vi "Main.vi"() -> ()   [LabVIEW 2015, in "Stock.lvlib"]
doc: "This template is based off of the Queued Message Handler design pattern and the Queued Message Handler project template that ships with LabVIEW.\n\nThe main difference is that the queue is private to this module and communication between modules is performed via Broadcast and Request events.\n\nRequest events are wrapped in public API methods and are handled in the Event Handling Loop (EHL) of this VI. Any module can register for Broadcast events sent by this module. The EHL generates messages based on user interface actions.\n\nThe Message Handling Loop (MHL) processes messages generated by the EHL, or by other messages. The messages are string values, so new messages can be added easily to the Message Cases case structure in the MHL. Each message cluster can also provide an optional value for Message Data, which is a variant that can be converted to whatever message-specific data is required.\n_____\nBased on Delacor QMH Project Template 4.2.1.64."
uses:
  Stock.lvlib
  <vilib>/Delacor/Delacor QMH/Libraries/Module Admin_class/Delacor_lib_QMH_Module Admin.lvclass
  Module Data--cluster.ctl
  Products.ctl
  <vilib>/Delacor/Delacor QMH/Libraries/Message Queue_class/Delacor_lib_QMH_Message Queue.lvclass/Delacor_lib_QMH_Message Queue.ctl
  Stop Argument--cluster.ctl
  <vilib>/Delacor/Delacor QMH/Libraries/Module Admin_class/Delacor_lib_QMH_Module Admin.lvclass/Delacor_lib_QMH_Module Admin.ctl
  In Stock and Price Argument--cluster.ctl
  In Stock and Price (Reply Payload)--cluster.ctl
  Reduce Stock Level Argument--cluster.ctl
  Reduce Stock Level (Reply Payload)--cluster.ctl
  <vilib>/Utility/miscctls.llb/LVPointTypeDef.ctl
  <vilib>/Delacor/Delacor QMH/Libraries/Message Queue_class/Delacor_lib_QMH_Enqueue Message (Single).vi
  <vilib>/Delacor/Delacor QMH/Libraries/Module Admin_class/Delacor_lib_QMH_Get External Launch.vi
  <vilib>/Utility/error.llb/Error Cluster From Error Code.vi
  <vilib>/ErrorRing/Error Ring.xnode
  <vilib>/Delacor/Delacor QMH/Libraries/Message Queue_class/Delacor_lib_QMH_Message Queue.lvclass
panel:
  in  "Subpanel Ref":refnum<vi>
  out "Stock Levels":T1(array[cluster]) {"Price" format="£%.2f"; "Stock Level" scale=0.0..58.0}
  in  "Simulate MHL Error":bool
  in  "Simulate EHL Error":bool
  out "error out":errorcluster
  in  "Module Admin":refnum<class "Delacor_lib_QMH_Module Admin.lvclass">
  out "Status":string
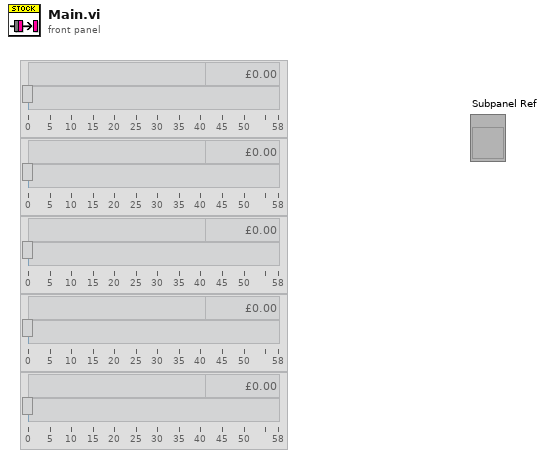
[diagram p1: front panel]
types:
  T1 = cluster{"Name":string, "Price":dbl, "Stock Level":dbl}[]
  T2 = typedef "Stock.lvlib/Request Events--cluster.ctl" = cluster{"Stop Module":refnum<user-event>, "Show Panel":refnum<user-event>, "Hide Panel":refnum<user-event>, "Get Module Execution Status":refnum<user-event>, "Show Diagram":refnum<user-event>, "In Stock and Price":refnum<user-event>, "Reduce Stock Level":refnum<user-event>}
  T3 = typedef "Stock.lvlib/Module Data--cluster.ctl" = cluster{"Status":string, "Stock":T4[], "Stock File Path":path}
  T4 = typedef "Stock.lvlib/Products.ctl" = cluster{"Name":string, "Price (pence/cents)":u32, "Stock Level":u32}
  T5 = enum32{"invalid lock state", "Not Locked", "Locked (No Password)", "Password-protected"}
  T6 = typedef "Stock.lvlib/Stop Argument--cluster.ctl" = cluster{"Origin":string, "Exit via Stop Module Req?":bool, "Wait for Module to stop?":bool}
  T7 = typedef "Stock.lvlib/In Stock and Price Argument--cluster.ctl" = cluster{"Stock Item":u32, "Wait Notifier":refnum<notifier>, "wait for reply":bool}
  T8 = typedef "Stock.lvlib/Reduce Stock Level Argument--cluster.ctl" = cluster{"Product":i32, "Wait Notifier":refnum<notifier>, "wait for reply":bool}
  T9 = typedef "LVPointTypeDef.ctl" = cluster{"Horizontal":i16, "Vertical":i16}
  T10 = typedef "Stock.lvlib/In Stock and Price (Reply Payload)--cluster.ctl" = cluster{"In Stock?":bool, "Price (Pence)":u32, "In Stock and Price_error":errorcluster}
  T11 = typedef "Stock.lvlib/Reduce Stock Level (Reply Payload)--cluster.ctl" = cluster{"Sucessful?":bool, "Reduce Stock Level_error":errorcluster}
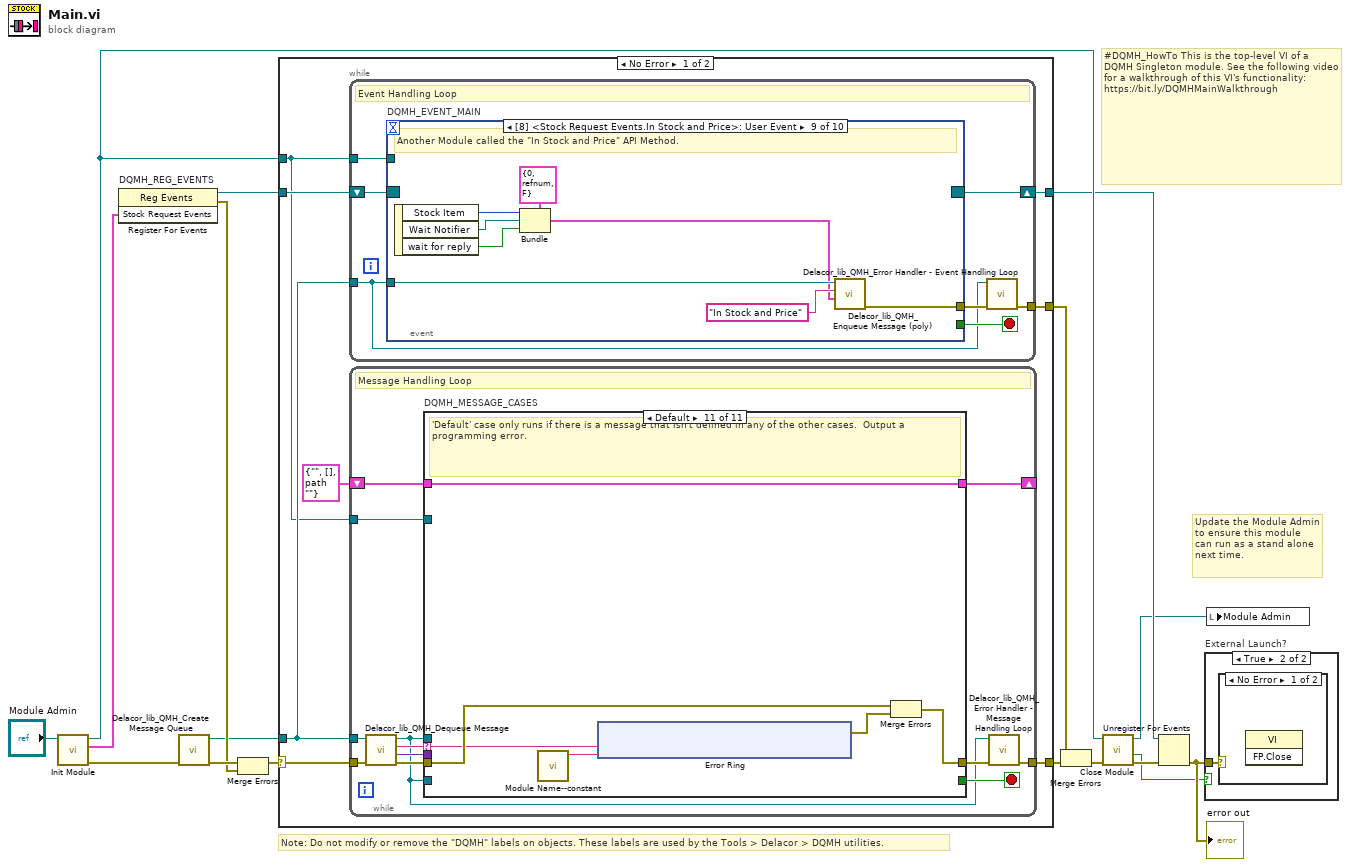
[diagram p0: block diagram]
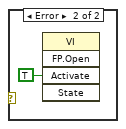
[diagram p3: hidden frame]
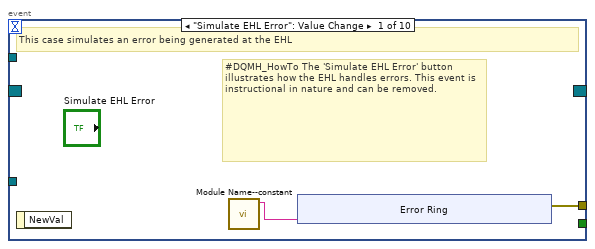
[diagram p4: hidden frame]
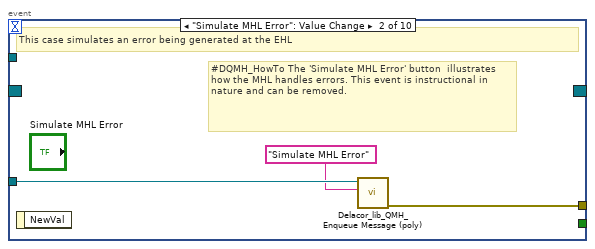
[diagram p5: hidden frame]
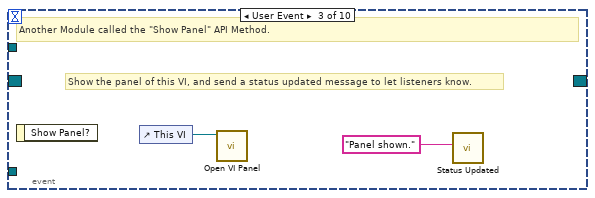
[diagram p6: hidden frame]
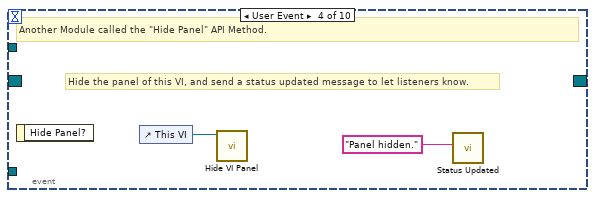
[diagram p7: hidden frame]
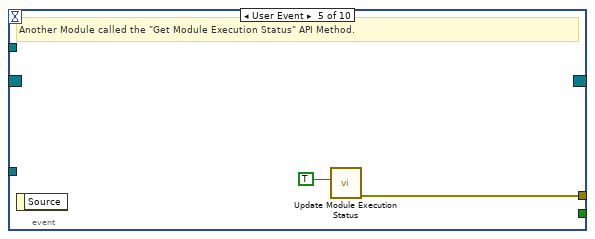
[diagram p8: hidden frame]
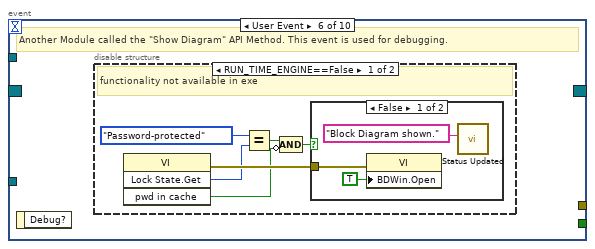
[diagram p9: hidden frame]
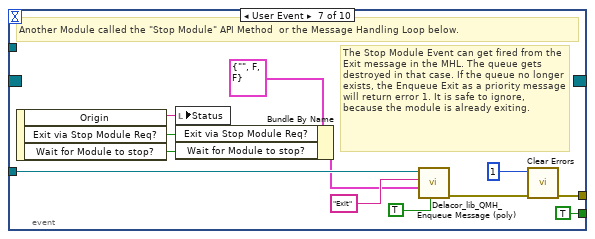
[diagram p12: hidden frame]
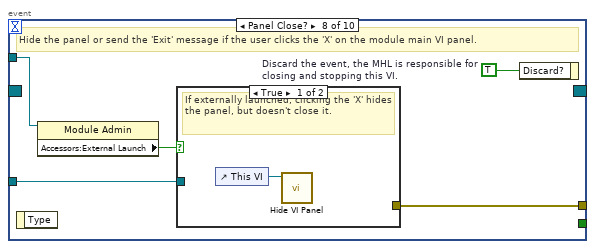
[diagram p13: hidden frame]
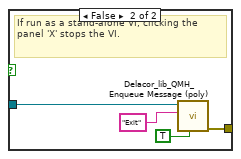
[diagram p14: hidden frame]
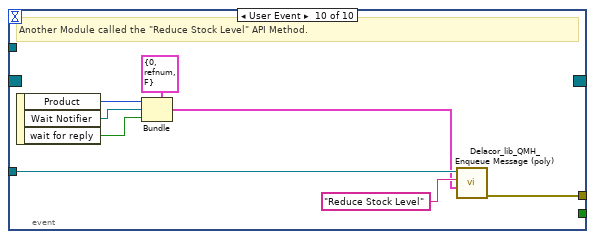
[diagram p15: hidden frame]
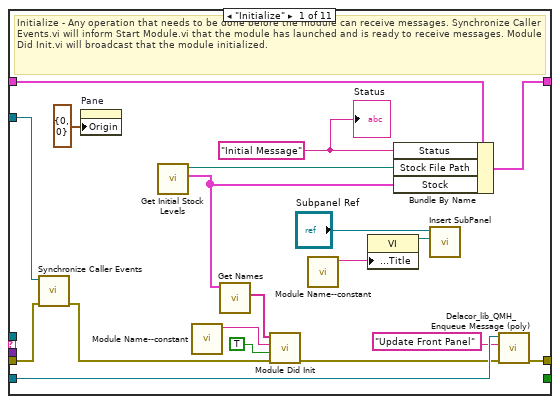
[diagram p16: hidden frame]
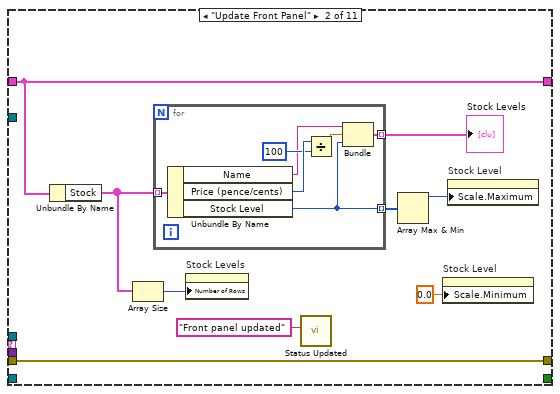
[diagram p17: hidden frame]
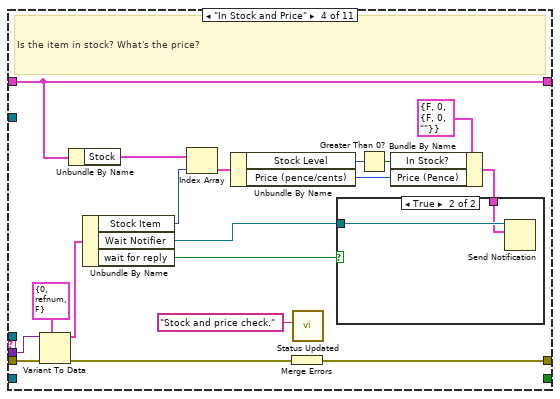
[diagram p19: hidden frame]
diagram:
  # "#DQMH_HowTo This is the top-level VI of a DQMH Singleton module. See the following video for a walkthrough of this VI's functionality: https://bit.ly/DQMHMainWalkthrough"
  # "Note: Do not modify or remove the \"DQMH\" labels on objects. These labels are used by the Tools > Delacor > DQMH utilities."
  # "Update the Module Admin to ensure this module can run as a stand alone next time."
  n1 = call "Init Module.vi"("Singleton Module Admin in"="Module Admin") -> ("error out"=w16:errorcluster, "Stock Request Events"=w5:T2, "Singleton Module Admin out"=w8:refnum<class "Delacor_lib_QMH_Module Admin.lvclass">)  [unwired: 8 in]
  n2 = register-events "DQMH_REG_EVENTS"(w5) -> (reference out=w6:refnum<event-registration>, error out=w9:errorcluster)  [unwired: 2 in]
  n3 = call <vilib>:"Delacor_lib_QMH_Create Message Queue.vi"("error in (no error)"=w16) -> ("error out"=w11:errorcluster, "Message Queue"=w4:refnum<class "Delacor_lib_QMH_Message Queue.lvclass">)  [unwired: 9 in]
  n4 = Merge Errors(w11, w9) -> (w10:errorcluster)
  n5 = case shown="No Error" w10 {
    selector: w10 -> [w23 w257]
    tunnel: [w25 w257] -> w17
    tunnel: [w22 w254] -> w7
    tunnel: w6 -> [w20 w254]
    tunnel: w4 -> [w19 _]
    tunnel: [w24 _] -> w14
    tunnel: w8 -> [w18 w250]
    frame No Error {
      n6 = while {
        tunnel: w19 -> [w26]
        shift-right: [w29] -> w22
        shift-left: w20 -> [w30]
        tunnel: [w31] -> w24
        tunnel: w18 -> [w27]
        stop <- w28 stop-if-true
        # "Event Handling Loop"
        n7 = event "DQMH_EVENT_MAIN" shown="[8] <Stock Request Events.In Stock and Price>: User Event" {
          selector: w30 -> [_ _ _ _ _ _ _ _ _ _]
          dyn-events: [_ _ _ _ _ _ _ _ _ _] -> w29
          timeout: _ -> [_ _ _ _ _ _ _ _ _ _]
          tunnel: [_ _ _ _ _ _ TRUE ("Discard?") _ _ _] -> w28
          tunnel: w26 -> [_ w43 _ _ _ _ w67 w74 w89 w97]
          tunnel: [w34 w44 _ _ w50 _ w70 w76 w82 w90] -> w32
          tunnel: w27 -> [_ _ _ _ _ _ _ w73 _ _]
          event "Simulate EHL Error": Value Change {
            # "#DQMH_HowTo The 'Simulate EHL Error' button  illustrates how the EHL handles errors. This event is instructional in nature and can be removed."
            # "This case simulates an error being generated at the EHL"
            n8 = event-data() -> ()  [unwired: 1 in, 1 out]
            n9 = call "Module Name--constant.vi"() -> ("Module Name"=w33:string)  [unwired: 11 in]
            n10 = xnode "Error Ring"("parameter 0"=w33) -> ("error out"=w34:errorcluster)
          }
          event "Simulate MHL Error": Value Change {
            # "#DQMH_HowTo The 'Simulate MHL Error' button  illustrates how the MHL handles errors. This event is instructional in nature and can be removed."
            # "This case simulates an error being generated at the EHL"
            n11 = event-data() -> ()  [unwired: 1 in, 1 out]
            n12 = call-poly <vilib>:"Delacor_lib_QMH_Enqueue Message (poly).vi"("Message"="Simulate MHL Error", "Message Queue in"=w43) -> ("error out"=w44:errorcluster)  [unwired: 8 in, 1 out]
          }
          event User Event {
            # "Show the panel of this VI, and send a status updated message to let listeners know."
            # "Another Module called the \"Show Panel\" API Method."
            n13 = event-data() -> ()  [unwired: 1 in, 1 out]
            n14 = control-ref of="This VI"() -> (w46:refnum<vi>)
            n15 = call "Open VI Panel.vi"("VI"=w46) -> ()  [unwired: 10 in, 1 out]
            n16 = call "Status Updated.vi"("Status"="Panel shown." ("format string")) -> ()  [unwired: 10 in, 1 out]
          }
          event User Event {
            # "Hide the panel of this VI, and send a status updated message to let listeners know."
            # "Another Module called the \"Hide Panel\" API Method."
            n17 = event-data() -> ()  [unwired: 1 in, 1 out]
            n18 = control-ref of="This VI"() -> (w48:refnum<vi>)
            n19 = call "Hide VI Panel.vi"("VI"=w48) -> ()  [unwired: 10 in, 1 out]
            n20 = call "Status Updated.vi"("Status"="Panel hidden." ("format string")) -> ()  [unwired: 10 in, 1 out]
          }
          event User Event {
            # "Another Module called the \"Get Module Execution Status\" API Method."
            n21 = event-data() -> ()  [unwired: 1 in, 1 out]
            n22 = call "Update Module Execution Status.vi"("Running?"=TRUE) -> ("error out"=w50:errorcluster)  [unwired: 10 in]
          }
          event User Event {
            # "Another Module called the \"Show Diagram\" API Method. This event is used for debugging."
            n23 = event-data() -> ()  [unwired: 1 in, 1 out]
            n24 = disable-structure shown="RUN_TIME_ENGINE==False" {
              frame condition #0 (active) {
                # "functionality not available in exe"
                n25 = invoke class="VI" method="Lock State.Get"() -> (error out=w56:errorcluster, "Get Lock State"=w55:T5, "pwd in cache"=w52:bool)  [unwired: 4 in, 1 out]
                n26 = Equal?(x=T5."Password-protected", y=w55) -> (x = y?=w53:bool)
                n27 = Compound Arithmetic op=AND(w53, invert w52) -> (w51:bool)
                n28 = case shown="False" w51 {
                  tunnel: w56 -> [w59 _]
                  frame False {
                    n29 = property class="VI"(error in=w59, "BDWin.Open"=TRUE ("Block Diagram Window:Open")) -> ()  [unwired: 1 in, 2 out]
                    n30 = call "Status Updated.vi"("Status"="Block Diagram shown." ("format string")) -> ()  [unwired: 10 in, 1 out]
                  }
                  frame True {
                    # "Password-protected VI, and the password is not in the cache. Do not show the diagram."
                  }
                }
              }
              frame condition #1 {
              }
            }
          }
          event User Event {
            # "The Stop Module Event can get fired from the Exit message in the MHL. The queue gets destroyed in that case. If the queue no longer exists, the Enqueue Exit as a priority message will return error 1. It is safe to ignore, because the module is already exiting."
            # "Another Module called the \"Stop Module\" API Method  or the Message Handling Loop below."
            n31 = event-data() -> ("Origin"=w66:string, "Exit via Stop Module Req?"=w62:bool, "Wait for Module to stop?"=w61:bool)  [unwired: 1 in]
            n32 = local write "Status"(w66) -> ()
            n33 = Bundle By Name(cluster=T6 {"Origin"="", "Exit via Stop Module Req?"=FALSE, "Wait for Module to stop?"=FALSE} ("Stop Argument"), "Exit via Stop Module Req?"=w62, "Wait for Module to stop?"=w61) -> (w60:T6)
            n34 = call-poly <vilib>:"Delacor_lib_QMH_Enqueue Message (poly).vi"("Priority Message? (F)"=TRUE, "Message Data"=w60, "Message"="Exit", "Message Queue in"=w67) -> ("error out"=w71:errorcluster)  [unwired: 6 in, 1 out]
            n35 = call <vilib>:"Clear Errors.vi"("error in (no error)"=w71, "specific error code to clear (0: all)"=1) -> ("error out"=w70:errorcluster)  [unwired: 4 in, 1 out]
          }
          event Panel Close? {
            w75 = TRUE  # Discard the event, the MHL is responsible for closing and stopping this VI.
            # "Hide the panel or send the 'Exit' message if the user clicks the 'X' on the module main VI panel."
            n36 = event-data() -> ()  [unwired: 1 in, 1 out]
            n37 = property class="Module Admin"(reference=w73) -> ("Accessors:External Launch"=w72:bool)  [unwired: 1 in, 2 out]
            n38 = case shown="True" w72 {
              tunnel: w74 -> [_ w80]
              tunnel: [_ w81] -> w76
              frame True {
                # "If externally launched, clicking the 'X' hides the panel, but doesn't close it."
                n39 = control-ref of="This VI"() -> (w77:refnum<vi>)
                n40 = call "Hide VI Panel.vi"("VI"=w77) -> ()  [unwired: 10 in, 1 out]
              }
              frame False {
                # "If run as a stand-alone VI, clicking the panel 'X' stops the VI."
                n41 = call-poly <vilib>:"Delacor_lib_QMH_Enqueue Message (poly).vi"("Priority Message? (F)"=TRUE, "Message"="Exit", "Message Queue in"=w80) -> ("error out"=w81:errorcluster)  [unwired: 7 in, 1 out]
              }
            }
            n42 = event-data("Discard?"=w75) -> ()  [unwired: 1 in, 1 out]
          }
          event User Event {
            # "Another Module called the \"In Stock and Price\" API Method."
            n43 = event-data() -> ("Stock Item"=w85:u32, "Wait Notifier"=w84:refnum<notifier>, "wait for reply"=w83:bool)  [unwired: 1 in]
            n44 = Bundle(cluster=T7 {"Stock Item"=0, "Wait Notifier"=refnum, "wait for reply"=FALSE} ("In Stock and Price Argument"), "Stock Item"=w85, "Wait Notifier"=w84, "wait for reply"=w83) -> (w86:T7)
            n45 = call-poly <vilib>:"Delacor_lib_QMH_Enqueue Message (poly).vi"("Message Data"=w86, "Message"="In Stock and Price", "Message Queue in"=w89) -> ("error out"=w82:errorcluster)  [unwired: 7 in, 1 out]
          }
          event User Event {
            # "Another Module called the \"Reduce Stock Level\" API Method."
            n46 = event-data() -> ("Product"=w93:i32, "Wait Notifier"=w92:refnum<notifier>, "wait for reply"=w91:bool)  [unwired: 1 in]
            n47 = Bundle(cluster=T8 {"Product"=0, "Wait Notifier"=refnum, "wait for reply"=FALSE} ("Reduce Stock Level Argument"), "Product"=w93, "Wait Notifier"=w92, "wait for reply"=w91) -> (w94:T8)
            n48 = call-poly <vilib>:"Delacor_lib_QMH_Enqueue Message (poly).vi"("Message Data"=w94, "Message"="Reduce Stock Level", "Message Queue in"=w97) -> ("error out"=w90:errorcluster)  [unwired: 7 in, 1 out]
          }
        }
        n49 = call-dynamic "Delacor_lib_QMH_Error Handler - Event Handling Loop.vi"("error in (no error)"=w32, "Message Queue in"=w26) -> ("dup error in"=w31:errorcluster)  [unwired: 8 in, 1 out]
      }
      n50 = while {
        tunnel: w19 -> [w100]
        shift-right: [w104] -> _
        shift-left: T3 {"Status"="", "Stock"=[], "Stock File Path"=path ""} ("Data Cluster") -> [w105]
        tunnel: w23 -> [w108]
        tunnel: [w106] -> w25
        tunnel: w18 -> [w99]
        stop <- w103 stop-if-true
        # "Message Handling Loop"
        n51 = call-dynamic "Delacor_lib_QMH_Dequeue Message.vi"("error in (no error)"=w108, "Message Queue in"=w100) -> ("error out"=w107:errorcluster, "Message Data"=w101:variant, "Message"=w102:string, "Message Queue out"=w98:refnum<class "Delacor_lib_QMH_Message Queue.lvclass">)  [unwired: 6 in]
        n52 = case "DQMH_MESSAGE_CASES" shown="Default" w102 {
          selector: w102 -> [_ _ _ _ _ _ _ _ _ _ w237]
          tunnel: w98 -> [_ _ _ _ _ _ _ _ w207 w229 _]
          tunnel: w107 -> [w128 w137 w146 w164 w185 w190 w192 w197 w214 w235 w239]
          tunnel: [w116 w137 w146 w155 w169 w189 w192 w196 w210 w232 w240] -> w109
          tunnel: w105 -> [w125 w136 w145 w154 w177 w188 w191 w194 w209 w228 w238]
          tunnel: [w124 w136 w145 w154 w176 w188 w191 w194 w209 w228 w238] -> w104
          tunnel: [_ _ _ _ _ _ _ _ _ w227 _] -> w103
          tunnel: w101 -> [_ _ _ w162 w184 _ _ _ w208 w226 _]
          tunnel: w99 -> [w126 _ _ _ _ _ _ _ w206 w221 _]
          tunnel: w98 -> [w119 _ _ _ w168 _ _ _ _ _ _]
          frame "Initialize" {
            w120 = "Initial Message" ("Initial Message")
            # "Initialize - Any operation that needs to be done before the module can receive messages. Synchronize Caller Events.vi will inform Start Module.vi that the module has launched and is ready to receive messages. Module Did Init.vi will broadcast that the module initialized."
            n53 = call "Synchronize Caller Events.vi"("error in (no error)"=w128, "Singleton Module Admin in"=w126) -> ("error out"=w127:errorcluster)  [unwired: 8 in, 1 out]
            n54 = property on="Pane" class="Pane"("Origin"=T9 {"Horizontal"=0, "Vertical"=0}) -> ()  [unwired: 2 in, 2 out]
            n55 = call "Get Initial Stock Levels.vi"() -> ("Stock"=w111:T4[], "Stock file path"=w110:path)  [unwired: 10 in]
            n56 = call "Module Name--constant.vi"() -> ("Module Name"=w122:string)  [unwired: 11 in]
            n57 = call "Get Names.vi"("Stock"=w111) -> ("Product Names"=w115:string[])  [unwired: 10 in]
            n58 = call "Module Did Init.vi"("error in (no error)"=w127, "Initialized?"=TRUE, "Origin"=w122, "Product Names"=w115) -> ("error out"=w117:errorcluster)  [unwired: 7 in]
            n59 = call "Module Name--constant.vi"() -> ("Module Name"=w114:string)  [unwired: 11 in]
            n60 = property class="VI"("Front Panel.Title"=w114) -> (reference out=w112:refnum<vi>)  [unwired: 2 in, 1 out]
            n61 = Bundle By Name(cluster=w125, "Status"=w120, "Stock File Path"=w110, "Stock"=w111) -> (w124:T3)
            n62 = call "Insert SubPanel.vi"("VI Ref"=w112, "Subpanel Ref"="Subpanel Ref") -> ()  [unwired: 9 in, 1 out]
            n63 = call-poly <vilib>:"Delacor_lib_QMH_Enqueue Message (poly).vi"("error in (no error)"=w117, "Message"="Update Front Panel" ("Initial Message"), "Message Queue in"=w119) -> ("error out"=w116:errorcluster)  [unwired: 7 in, 1 out]
            "Status" <- w120
          }
          frame "Update Front Panel" {
            n64 = Unbundle By Name(w136) -> ("Stock"=w132:T4[])
            n65 = Array Size(array=w132) -> (size(s)=w131:i32)
            n66 = for {
              tunnel: w132 -> [w144] mode=indexing
              tunnel: [w141] -> w134 mode=indexing
              tunnel: [w138] -> w135 mode=indexing
              n67 = Unbundle By Name(w144) -> ("Name"=w139:string, "Price (pence/cents)"=w143:u32, "Stock Level"=w141:u32)
              n68 = Divide(x=w143, y=u32 100) -> (x/y=w140:dbl)
              n69 = Bundle("Name"=w139, w140, "Stock Level"=w141) -> (w138:cluster{"Name":string, dbl, "Stock Level":u32})  [unwired: 1 in]
            }
            "Stock Levels" <- w135
            n70 = property on="Stock Levels" class="Arr (strict)"("Number of Rows"=w131) -> ()  [unwired: 2 in, 2 out]
            n71 = call "Status Updated.vi"("Status"="Front panel updated") -> ()  [unwired: 10 in, 1 out]
            n72 = Array Max & Min(array=w134) -> (max value=w133:u32)  [unwired: 3 out]
            n73 = property on="Stock Level" class="Slide (strict)"("Scale.Minimum"=0.0 ("Scale.Range:Minimum")) -> ()  [unwired: 2 in, 2 out]
            n74 = property on="Stock Level" class="Slide (strict)"("Scale.Maximum"=w133) -> ()  [unwired: 2 in, 2 out]
          }
          frame "--- Module Specific ---" {
            # "Separator -- The following cases handle messages specific to this Module."
          }
          frame "In Stock and Price" {
            # "Is the item in stock? What's the price?"
            n75 = Variant To Data(error in=w164, type=T7 {"Stock Item"=0, "Wait Notifier"=refnum, "wait for reply"=FALSE} ("In Stock and Price Argument"), Variant=w162) -> (data=w160:T7, error out=w163:errorcluster)
            n76 = Unbundle By Name(w154) -> ("Stock"=w153:T4[])
            n77 = Unbundle By Name(w160) -> ("Stock Item"=w152:u32, "Wait Notifier"=w159:refnum<notifier>, "wait for reply"=w158:bool)
            n78 = Index Array(array=w153, index=w152) -> (element=w151:T4)
            n79 = Unbundle By Name(w151) -> ("Stock Level"=w149:u32, "Price (pence/cents)"=w150:u32)
            n80 = Merge Errors(w163) -> (w155:errorcluster)
            n81 = call "Status Updated.vi"("Status"="Stock and price check.") -> ()  [unwired: 10 in, 1 out]
            n82 = Greater Than 0?(x=w149) -> (x > 0?=w148:bool)
            n83 = Bundle By Name(cluster=T10 {"In Stock?"=FALSE, "Price (Pence)"=0, "In Stock and Price_error"={"status"=FALSE, "code"=0, "source"=""}} ("In Stock and Price (Reply Payload)"), "In Stock?"=w148, "Price (Pence)"=w150) -> (w157:T10)
            n84 = case shown="True" w158 {
              tunnel: w159 -> [_ w166]
              tunnel: w157 -> [_ w165]
              frame False {
              }
              frame True {
                n85 = Send Notification(notification=w165, notifier=w166) -> ()  [unwired: 1 in, 2 out]
              }
            }
          }
          frame "Reduce Stock Level" {
            # "Reduce the stock level and make sure it was sucessful."
            n86 = Variant To Data(error in=w185, type=T8 {"Product"=0, "Wait Notifier"=refnum, "wait for reply"=FALSE} ("Reduce Stock Level Argument"), Variant=w184) -> (data=w182:T8, error out=w173:errorcluster)
            n87 = Unbundle By Name(w182) -> ("Product"=w175:i32, "Wait Notifier"=w181:refnum<notifier>, "wait for reply"=w180:bool)
            n88 = call "Status Updated.vi"("Status"="Reducing stock level") -> ()  [unwired: 10 in, 1 out]
            n89 = call "Reduce Stock Level and Check.vi"("error in (no error)"=w173, "Product Index"=w175, "Data Cluster"=w177) -> ("error out"=w172:errorcluster, "Sucessful"=w174:bool, "Data Cluster Out"=w176:T3)  [unwired: 6 in]
            n90 = Merge Errors(w172) -> (w170:errorcluster)
            n91 = Bundle By Name(cluster=T11 {"Sucessful?"=FALSE, "Reduce Stock Level_error"={"status"=FALSE, "code"=0, "source"=""}} ("Reduce Stock Level (Reply Payload)"), "Sucessful?"=w174) -> (w179:T11)
            n92 = case shown="True" w180 {
              tunnel: w181 -> [_ w187]
              tunnel: w179 -> [_ w186]
              frame False {
              }
              frame True {
                n93 = Send Notification(notification=w186, notifier=w187) -> ()  [unwired: 1 in, 2 out]
              }
            }
            n94 = call-poly <vilib>:"Delacor_lib_QMH_Enqueue Message (poly).vi"("error in (no error)"=w170, "Message"="Update Front Panel" ("Initial Message"), "Message Queue in"=w168) -> ("error out"=w169:errorcluster)  [unwired: 7 in, 1 out]
          }
          frame "---Copy This Frame---" {
            # "Duplicate this frame when creating new messages.  Change this comment in the duplicated frame to describe this message."
            n95 = Merge Errors(w190) -> (w189:errorcluster)
          }
          frame "--- Exit and Error Handling---" {
            # "Separator - The following cases handle errors and exit messages."
          }
          frame "Simulate MHL Error" {
            # "#DQMH_HowTo The 'Simulate MHL Error' button  illustrates how the MHL handles errors. This event is instructional in nature and can be removed."
            # "Simulate an error occurring at the MHL"
            n96 = call "Module Name--constant.vi"() -> ("Module Name"=w193:string)  [unwired: 11 in]
            n97 = xnode "Error Ring"("parameter 0"=w193) -> ("error out"=w195:errorcluster)
            n98 = Merge Errors(w197, w195) -> (w196:errorcluster)
          }
          frame "Error" {
            # "#CodeRecommended - If you ever change the name of this \"Error\" message, you'll need to update the name in the Check Loop Error.vi as well."
            # "#CodeRecommended - If the module is running in standalone mode (External Launch = FALSE), this code will pop up an error dialog and call the 'Exit' message if an error occurs. Add more fine-grained error handling here."
            # "Error - Check the error message data and respond accordingly. This message is sent by the \"Error Handler\" VIs at the end of each loop in this application."
            n99 = property class="Module Admin"(reference=w206) -> ("Accessors:External Launch"=w205:bool)  [unwired: 1 in, 2 out]
            n100 = Variant To Data(error in=w214, type=errorcluster {"status"=FALSE, "code"=0, "source"=""} ("error constant"), Variant=w208) -> (data=w215:errorcluster, error out=w212:errorcluster)
            n101 = call "Error Reported.vi"("Error"=w215) -> ()  [unwired: 10 in, 1 out]
            n102 = case shown="True" w205 {
              tunnel: [w220 _] -> w211
              tunnel: w207 -> [w218 _]
              tunnel: w215 -> [w219 _]
              frame False {
                # "If the module is running standalone, then pop up an error dialog and call the \"Exit\" message."
                n103 = call <vilib>:"Simple Error Handler.vi"("error in (no error)"=w219) -> ()  [unwired: 4 in, 5 out]
                n104 = call-poly <vilib>:"Delacor_lib_QMH_Enqueue Message (poly).vi"("Priority Message? (F)"=TRUE, "Message"="Exit", "Message Queue in"=w218) -> ("error out"=w220:errorcluster)  [unwired: 7 in, 1 out]
              }
              frame True {
                # "If the module was launched externally, calling the Error Reported broadcast VI is the only action performed by the \"Error\" message. The module's caller can then process the error appropriately."
              }
            }
            n105 = Merge Errors(w212, w211) -> (w210:errorcluster)
            n106 = local write "error out"(w210) -> ()
          }
          frame "Exit" {
            w225 = 91  # 91: not all Exit messages will have an argument
            w227 = TRUE  # Stop the VI
            # "Release the message queue reference"
            # "#CodeNeeded - Add any required cleanup code here"
            # "Exit - Exit the application."
            n107 = Variant To Data(error in=w235, type=T6 {"Origin"="", "Exit via Stop Module Req?"=FALSE, "Wait for Module to stop?"=FALSE} ("Stop Argument"), Variant=w226) -> (data=w223:T6, error out=w231:errorcluster)
            n108 = call <vilib>:"Clear Errors.vi"("error in (no error)"=w231, "specific error code to clear (0: all)"=w225) -> ("error out"=w234:errorcluster)  [unwired: 4 in, 1 out]
            n109 = control-ref of="This VI"() -> (w222:refnum<vi>)
            n110 = call-dynamic "Delacor_lib_QMH_Release Message Queue.vi"("error in (no error)"=w234, "Message Queue"=w229) -> ("error out"=w233:errorcluster)  [unwired: 9 in]
            n111 = call "Handle Exit.vi"("Stop Argument"=w223, "Admin in"=w221, "VI reference"=w222) -> ("error out"=w230:errorcluster)  [unwired: 7 in, 1 out]
            n112 = Merge Errors(w233, w230) -> (w232:errorcluster)
          }
          frame Default {
            # "'Default' case only runs if there is a message that isn't defined in any of the other cases.  Output a programming error."
            n113 = call "Module Name--constant.vi"() -> ("Module Name"=w236:string)  [unwired: 11 in]
            n114 = xnode "Error Ring"("parameter 0"=w237, "parameter 1"=w236) -> ("error out"=w241:errorcluster)
            n115 = Merge Errors(w239, w241) -> (w240:errorcluster)
          }
        }
        n116 = call-dynamic "Delacor_lib_QMH_Error Handler - Message Handling Loop.vi"("error in (no error)"=w109, "Message Queue in"=w98) -> ("dup error in"=w106:errorcluster)  [unwired: 8 in, 1 out]
      }
    }
    frame Error {
      # "Synchronize Caller Events.vi will inform Start Module.vi that the module has launched and will let the code calling Start Module.vi register for broadcasts and would permit the caller receive the broadcast that an error occurred at launch time."
      n117 = call "Synchronize Caller Events.vi"("Singleton Module Admin in"=w250) -> ("error out"=w255:errorcluster)  [unwired: 9 in, 1 out]
      n118 = call "Module Name--constant.vi"() -> ("Module Name"=w253:string)  [unwired: 11 in]
      n119 = Format Into String(format string="An error occurred during initialization. %s is no longer running.", w253) -> (resulting string=w251:string)  [unwired: 2 in, 1 out]
      n120 = Merge Errors(w257, w255) -> (w256:errorcluster)
      n121 = call "Error Reported.vi"("Additional Information"=w251, "Error"=w256) -> ()  [unwired: 9 in, 1 out]
    }
  }
  n122 = Merge Errors(w14, w17) -> (w13:errorcluster)
  n123 = call "Close Module.vi"("error in (no error)"=w13, "Module Admin in"=w8) -> ("error out"=w15:errorcluster, "External Launch"=w1:bool, "Module Admin out"=w2:refnum<class "Delacor_lib_QMH_Module Admin.lvclass">)  [unwired: 7 in]
  n124 = Unregister For Events(event registration refnum=w7, error in=w15) -> (error out=w12:errorcluster)
  "error out" <- w12
  n125 = case "External Launch?" shown="True" w1 {
    tunnel: w12 -> [_ w258]
    frame False {
    }
    frame True {
      n126 = case shown="No Error" w258 {
        frame No Error {
          n127 = invoke class="VI" method="FP.Close"() -> ()  [unwired: 3 in, 3 out]
        }
        frame Error {
          n128 = invoke class="VI" method="FP.Open"("Activate"=TRUE ("Activate?")) -> ()  [unwired: 4 in, 5 out]
        }
      }
    }
  }
  n129 = local write "Module Admin"(w2) -> ()
